vi "PCO_Storage.vi"() -> (0 "PCO_Storage":T1, 1 "PCO_Storage_Raw":T2, 2 "Length":u16, 3 "Raw_Length":u16)   [LabVIEW 2019, in "SDK.lvlib" / "Structures.lvlib"]
doc: "Use this template to build a VI to use as a subVI."
uses:
  Structures.lvlib
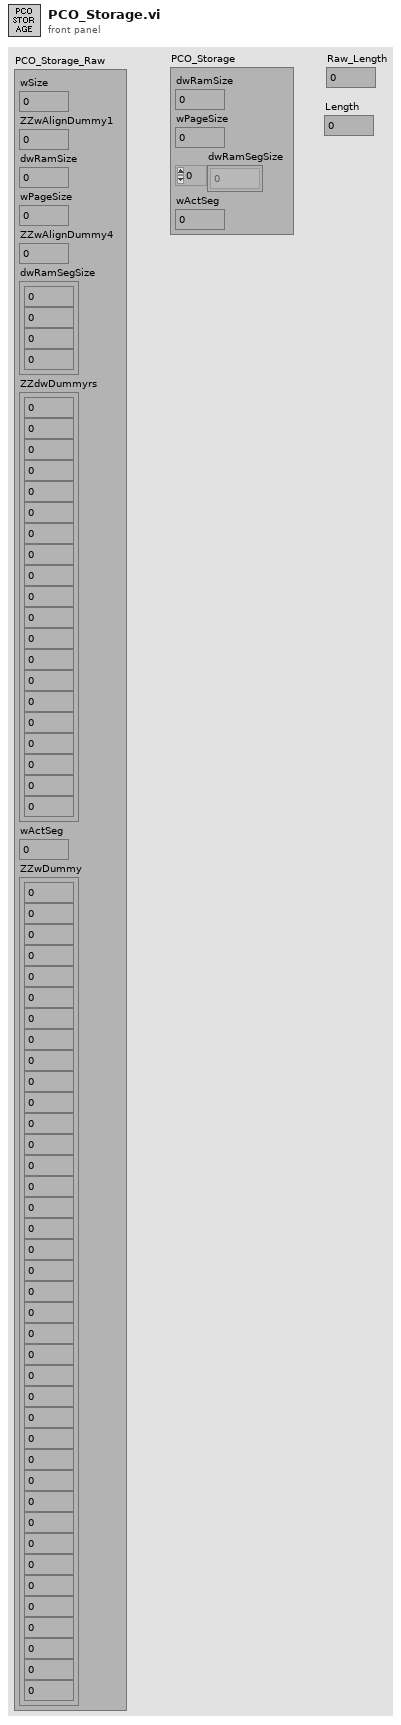
[diagram p1: front panel]
types:
  T1 = cluster{"dwRamSize":u32, "wPageSize":u16, "dwRamSegSize":u32[], "wActSeg":u16}
  T2 = cluster{"wSize":u16, "ZZwAlignDummy1":u16, "dwRamSize":u32, "wPageSize":u16, "ZZwAlignDummy4":u16, "dwRamSegSize":cluster{u32, u32, u32, u32}, "ZZdwDummyrs":cluster{u32, u32, u32, u32, u32, u32, u32, u32, u32, u32, u32, u32, u32, u32, u32, u32, u32, u32, u32, u32}, "wActSeg":u16, "ZZwDummy":cluster{u16, u16, u16, u16, u16, u16, u16, u16, u16, u16, u16, u16, u16, u16, u16, u16, u16, u16, u16, u16, u16, u16, u16, u16, u16, u16, u16, u16, u16, u16, u16, u16, u16, u16, u16, u16, u16, u16, u16}}
  T3 = cluster{u16, u16, u16, u16, u16, u16, u16, u16, u16, u16, u16, u16, u16, u16, u16, u16, u16, u16, u16, u16, u16, u16, u16, u16, u16, u16, u16, u16, u16, u16, u16, u16, u16, u16, u16, u16, u16, u16, u16}
  T4 = cluster{u32, u32, u32, u32, u32, u32, u32, u32, u32, u32, u32, u32, u32, u32, u32, u32, u32, u32, u32, u32}
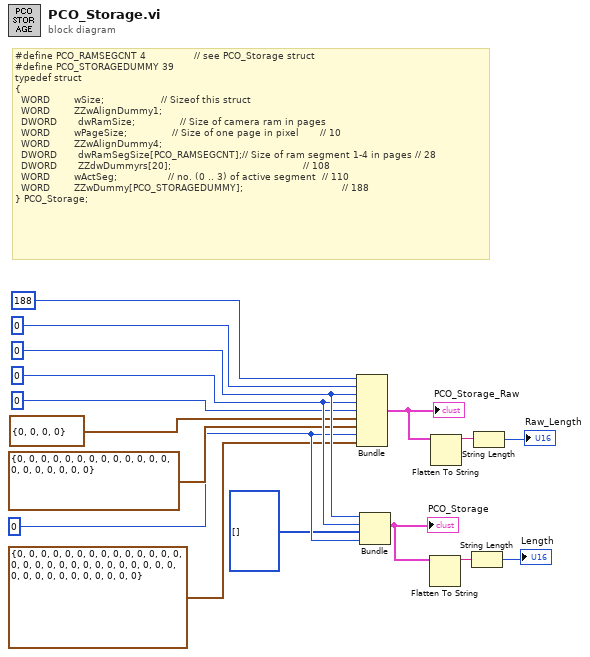
[diagram p0: block diagram]
diagram:
  w3 = u16 0 ("wActSeg")
  w7 = u16 0 ("wPageSize")
  w8 = u32 0 ("dwRamSize")
  # "#define PCO_RAMSEGCNT 4                // see PCO_Storage struct\n#define PCO_STORAGEDUMMY 39\ntypedef struct\n{\n  WORD        wSize;                   // Sizeof this struct\n  WORD        ZZwAlignDummy1;\n  DWORD       dwRamSize;               // Size of camera ram in pages\n  WORD        wPageSize;               // Size of one page in pixel       // 10\n  WORD        ZZwAlignDummy4;\n  DWORD       dwRamSegSize[PCO_RAMSEGCNT];// Size of ram segment 1-4 in pages // 28\n  DWORD       ZZdwDummyrs[20];                                            // 108\n  WORD        wActSeg;                 // no. (0 .. 3) of active segment  // 110\n  WORD        ZZwDummy[PCO_STORAGEDUMMY];                                 // 188\n} PCO_Storage;"
  n1 = Bundle("wSize"=u16 188, "ZZwAlignDummy1"=u16 0, "dwRamSize"=w8, "wPageSize"=w7, "ZZwAlignDummy4"=u16 0, "dwRamSegSize"=cluster{u32, u32, u32, u32} {0, 0, 0, 0}, "ZZdwDummyrs"=T4 {0, 0, 0, 0, 0, 0, 0, 0, 0, 0, 0, 0, 0, 0, 0, 0, 0, 0, 0, 0}, "wActSeg"=w3, "ZZwDummy"=T3 {0, 0, 0, 0, 0, 0, 0, 0, 0, 0, 0, 0, 0, 0, 0, 0, 0, 0, 0, 0, 0, 0, 0, 0, 0, 0, 0, 0, 0, 0, 0, 0, 0, 0, 0, 0, 0, 0, 0}) -> (w10:T2)  [unwired: 1 in]
  "PCO_Storage_Raw" <- w10
  n2 = Bundle("dwRamSize"=w8, "wPageSize"=w7, "dwRamSegSize"=u32[] [], "wActSeg"=w3) -> (w16:T1)  [unwired: 1 in]
  "PCO_Storage" <- w16
  n3 = Flatten To String(anything=w16) -> (data string=w15:string)  [unwired: 3 in, 2 out]
  n4 = Flatten To String(anything=w10) -> (data string=w14:string)  [unwired: 3 in, 2 out]
  n5 = String Length(string=w15) -> (length=→"Length":i32)
  n6 = String Length(string=w14) -> (length=→"Raw_Length":i32)
